vi "Read Attributes.vi"(11 "Resynchronize Microgrid Msg":refnum<class "Resynchronize Microgrid Msg.lvclass">) -> (2 "Payload":cluster{"Data":variant})   [LabVIEW 2018, in "Remote Operation Abstract.lvlib" / "Resynchronize Microgrid Msg.lvclass"]
uses:
  Resynchronize Microgrid Msg.lvclass
  Resynchronize Microgrid Msg.lvclass/Resynchronize Microgrid Msg.ctl
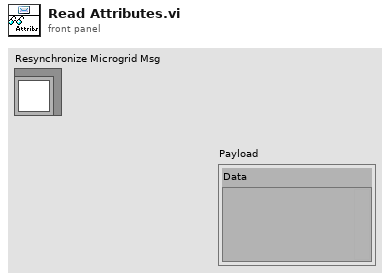
[diagram p1: front panel]
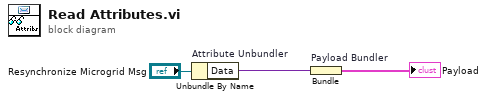
[diagram p0: block diagram]
diagram:
  n1 = Unbundle By Name "Attribute Unbundler"("Resynchronize Microgrid Msg") -> ("Data"=w1:variant)
  n2 = Bundle "Payload Bundler"("Data"=w1) -> (→"Payload":cluster{"Data":variant})  [unwired: 1 in]
